vi "Reset Tag.vi"(7 "Tree In":refnum<class "Tree.lvclass">, 8 "error in (no error)":errorcluster, 9 "New Tag":string, 10 "Original Tag":string, 11 "Composite Tree Data in":refnum<class "Composite Tree Data.lvclass">) -> (0 "error out":errorcluster, 3 "Composite Tree Data out":refnum<class "Composite Tree Data.lvclass">, 5 "Tree Out":refnum<class "Tree.lvclass">)   [LabVIEW 2024, in "Composite Tree Data.lvclass"]
uses:
  Composite Tree Data.lvclass
  Tree/Tree.lvclass
  Composite Tree Data.lvclass/Composite Tree Data.ctl
  Tree Data/Tree Data.lvclass/Tree Data.ctl
  Tree Data/Protected Data/Read Tag.vi
  Tree Data/Tree Data.lvclass
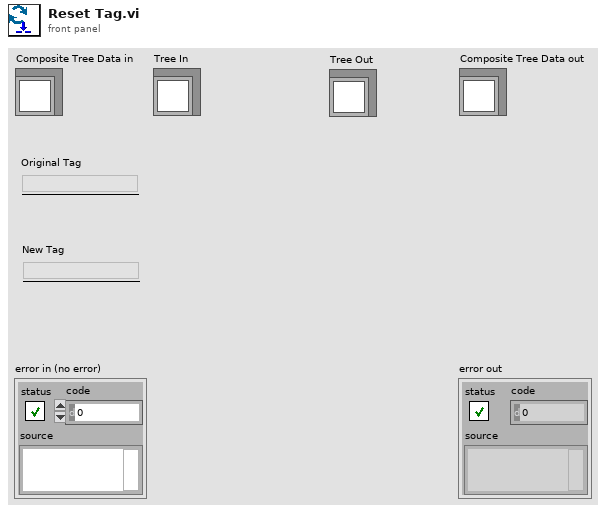
[diagram p1: front panel]
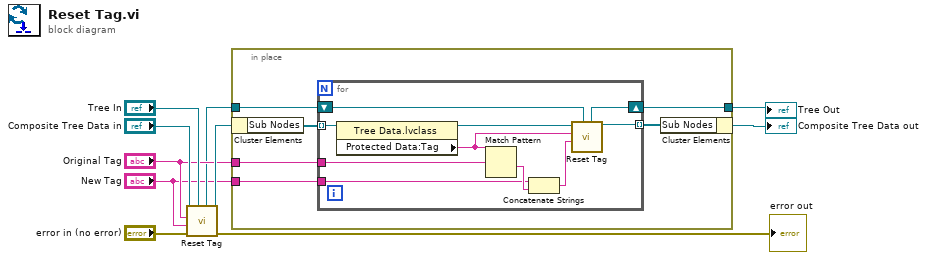
[diagram p0: block diagram]
diagram:
  n1 = call-parent "Reset Tag.vi"("Tree In"="Tree In", "error in (no error)"="error in (no error)", "New Tag"="New Tag", "Original Tag"="Original Tag", "Tree Data in"="Composite Tree Data in") -> ("error out"=→"error out":errorcluster, "Tree Data out"=w6:refnum<class "Composite Tree Data.lvclass">, "Tree Out"=w3:refnum<class "Tree.lvclass">)  [unwired: 4 in]
  n2 = in-place {
    in-place-border: "Original Tag" -> [w15]
    in-place-border: w3 -> [w13]
    in-place-border: "New Tag" -> [w12]
    in-place-border: [w11] -> w1
    n3 = in-place-cluster #1(w6) -> ("Sub Nodes"=w16:refnum<class "Tree Data.lvclass">[])
    n4 = for {
      tunnel: w16 -> [w25] mode=indexing
      tunnel: w15 -> [w22]
      tunnel: [w26] -> w14 mode=indexing
      shift-right: [w20] -> w11
      shift-left: w13 -> [w23]
      tunnel: w12 -> [w18]
      n5 = property class="Tree Data.lvclass"(reference=w25) -> (reference out=w24:refnum<class "Tree Data.lvclass">, "Protected Data:Tag"=w21:string)  [unwired: 1 in, 1 out]
      n6 = Match Pattern(string=w21, regular expression=w22) -> (after substring=w19:string)  [unwired: 1 in, 3 out]
      n7 = Concatenate Strings(w18, w19) -> (w17:string)
      n8 = call-dynamic "Reset Tag.vi"("Tree In"=w23, "New Tag"=w17, "Original Tag"=w21, "Tree Data in"=w24) -> ("Tree Data out"=w26:refnum<class "Tree Data.lvclass">, "Tree Out"=w20:refnum<class "Tree.lvclass">)  [unwired: 5 in, 1 out]
    }
    n9 = in-place-cluster #1("Sub Nodes"=w14) -> (→"Composite Tree Data out":refnum<class "Composite Tree Data.lvclass">)
  }
  "Tree Out" <- w1
